vi "Pump waveplate.vi"(4 "Axis in":i32=3, 5 "Trigger rate warnings?":bool, 6 "appended array":dbl[][](array[numeric]), 7 "Trigger rate \nat 52.6 degrees":dbl, 8 "error in (no error)":errorcluster, 9 "Photon #":i32, 10 "Target trial \nlength (ms)":dbl, 11 "VISA Refnum in":refnum<visa-resource-name>) -> (0 "error out":errorcluster, 1 "WP Error":bool=TRUE, 2 "Current position (units)":dbl, 3 "VISA Refnum out":refnum<visa-resource-name>)   [LabVIEW 2013]
uses:
  <vilib>/imath/engines/lvmath2/RunTimeEngine/BuiltInFunctions/asin/NIMS_asin(C).vi
  <instcachedir>/0/NIMS_asin(C)_73B68F6B04904A8785972686F67E90FD.lvgen/NIMS_asin(C)_73B68F6B04904A8785972686F67E90FD_001.vi
  <vilib>/imath/engines/lvmath2/RunTimeEngine/NodeEndStatement/NIMS_NodeEndStatement_Output.vi
  <instcachedir>/0/NIMS_NodeEndStatement_Output_53EC0D466D134D7ABD903AC30B43404B.lvgen/NIMS_NodeEndStatement_Output_53EC0D466D134D7ABD903AC30B43404B_010.vi
  <instcachedir>/0/NIMS_NodeEndStatement_Output_53EC0D466D134D7ABD903AC30B43404B.lvgen/NIMS_NodeEndStatement_Output_53EC0D466D134D7ABD903AC30B43404B_001.vi
  <vilib>/imath/engines/lvmath2/RunTimeEngine/BuiltInFunctions/abs/NIMS_abs(signed).vi
  <instcachedir>/0/NIMS_abs(signed)_C4FCB8E6058B49B797C7C8D53CA5F6EC.lvgen/NIMS_abs(signed)_C4FCB8E6058B49B797C7C8D53CA5F6EC_000.vi
  <vilib>/imath/engines/lvmath2/RunTimeEngine/ErrorHandling/NIMS_Finalize Error.vi
  <instcachedir>/0/NIMS_NodeEndStatement_Output_53EC0D466D134D7ABD903AC30B43404B.lvgen/NIMS_NodeEndStatement_Output_53EC0D466D134D7ABD903AC30B43404B_009.vi
  <instcachedir>/0/NIMS_abs(signed)_C4FCB8E6058B49B797C7C8D53CA5F6EC.lvgen/NIMS_abs(signed)_C4FCB8E6058B49B797C7C8D53CA5F6EC_002.vi
panel:
  out "angle":dbl
  out "theta1":dbl
  out "t_ratio":dbl
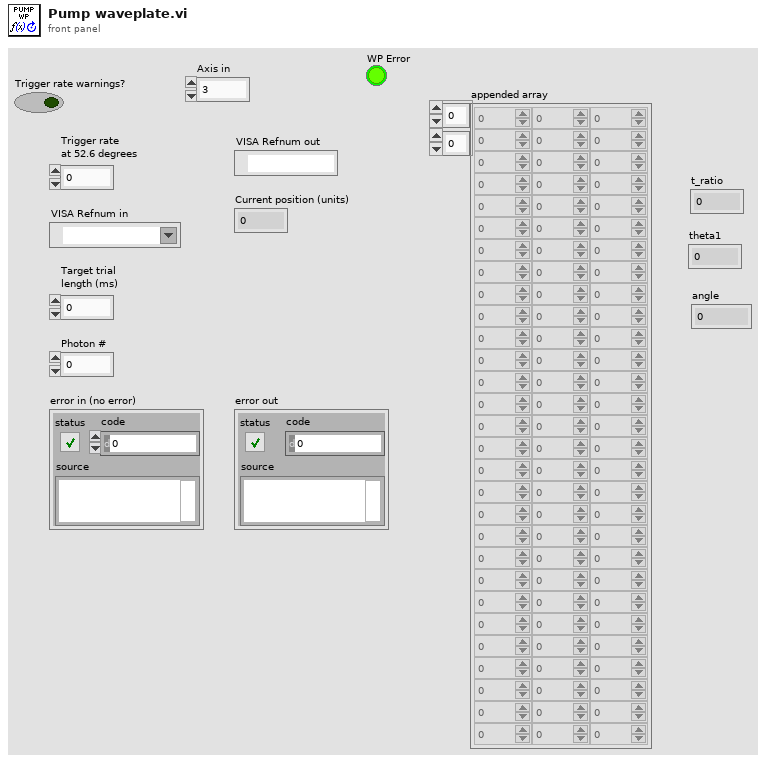
[diagram p1: front panel]
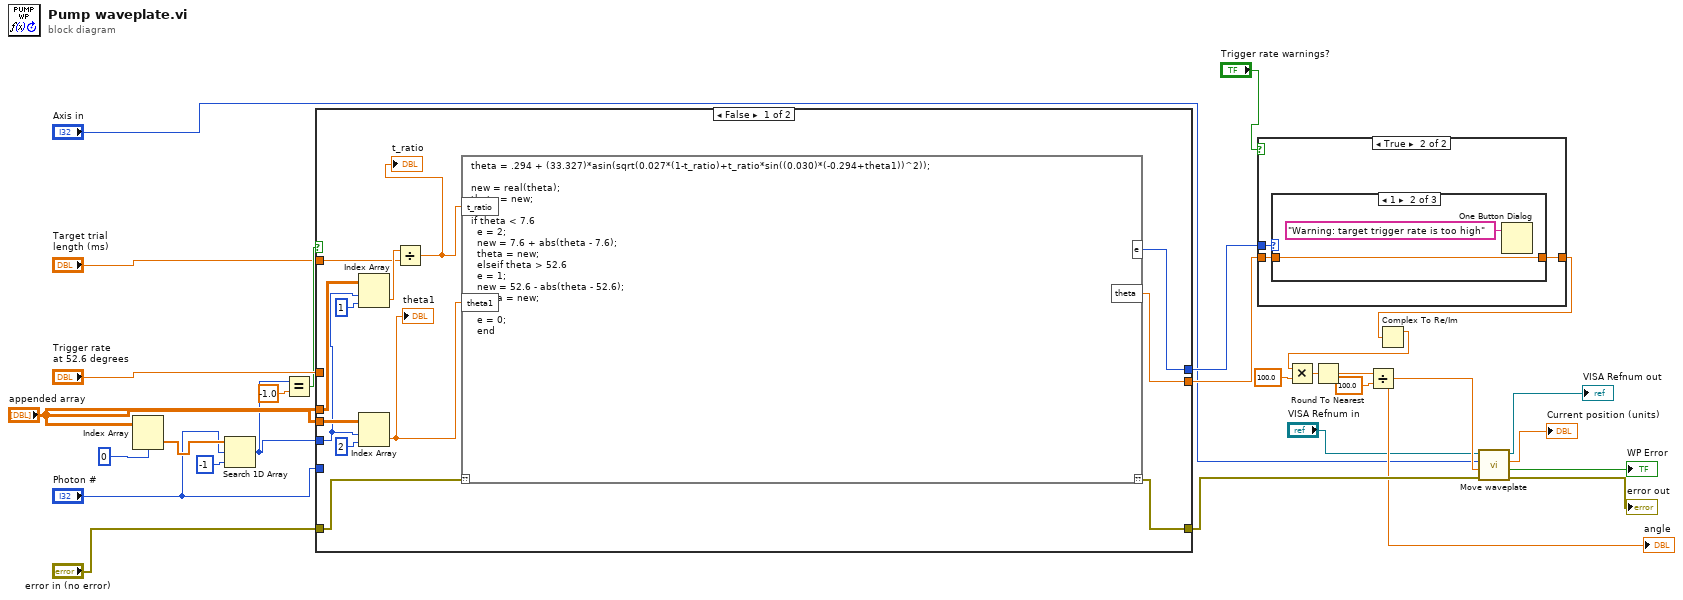
[diagram p0: block diagram]
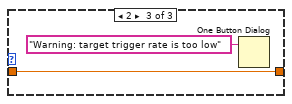
[diagram p4: hidden frame]
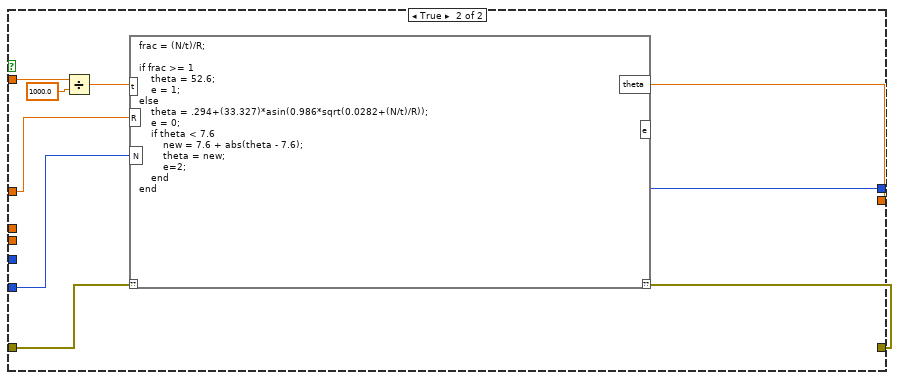
[diagram p5: hidden frame]
diagram:
  n1 = Index Array(array="appended array", index (col)=0 ("disabled index (col)")) -> (element=w24:dbl[])  [unwired: 1 in]
  n2 = Search 1D Array(1D array=w24, element="Photon #", start index (0)=-1) -> (index of element=w19:i32)
  n3 = Equal?(x=w19, y=-1.0) -> (x = y?=w21:bool)
  n4 = case shown="False" w21 {
    tunnel: "Trigger rate \nat 52.6 degrees" -> [_ w177]
    tunnel: [w29 w169] -> w16
    tunnel: [w32 w176] -> w27
    tunnel: "Target trial \nlength (ms)" -> [w33 w171]
    tunnel: "Photon #" -> [_ w175]
    tunnel: "error in (no error)" -> [w31 w174]
    tunnel: [w30 w173] -> w8
    tunnel: "appended array" -> [w36 _]
    tunnel: "appended array" -> [w35 _]
    tunnel: w19 -> [w34 _]
    frame False {
      n5 = Index Array(array=w35, index (row)=w34, index (col)=1 ("disabled index (col)")) -> (element=w39:dbl)
      n6 = Index Array(array=w36, index (row)=w34, index (col)=2 ("disabled index (col)")) -> (element=w38:dbl)
      "theta1" <- w38
      n7 = Divide(x=w39, y=w33) -> (x/y=w37:dbl)
      "t_ratio" <- w37
      n8 = mathscript code="theta = .294 + (33.327)*asin(sqrt(0.027*(1-t_ratio)+t_ratio*sin((0.030)*(-0.294+theta1))^2));\n\nnew = real(theta);\ntheta = new;\n\nif theta < 7.6\n  e = 2;\n  new = 7.6 + abs(theta - 7.6);\n  theta = new;\n  elseif theta > 52.6\n  e = 1;\n  new = 52.6 - abs(theta - 52.6);\n  theta = new;\n  else\n  e = 0;\n  end"("??"=w31, "t_ratio"=w37, "theta1"=w38) -> ("??"=w30:errorcluster, "e"=w32:i32, "theta"=w29:dbl)
    }
    frame True {
      n9 = Divide(x=w171, y=1000.0) -> (x/y=w170:dbl)
      n10 = mathscript code="frac = (N/t)/R;\n\nif frac >= 1\n    theta = 52.6;\n    e = 1;\nelse\n    theta = .294+(33.327)*asin(0.986*sqrt(0.0282+(N/t)/R));\n    e = 0;\n    if theta < 7.6\n        new = 7.6 + abs(theta - 7.6);\n        theta = new;\n        e=2;\n    end\nend"("??"=w174, "t"=w170, "R"=w177, "N"=w175) -> ("??"=w173:errorcluster, "e"=w176:i32, "theta"=w169:cdb)
    }
  }
  n11 = case shown="True" "Trigger rate warnings?" {
    tunnel: [w294 w297] -> w15
    tunnel: w16 -> [w294 w296]
    tunnel: w27 -> [_ w295]
    frame False {
    }
    frame True {
      n12 = case shown="1" w295 {
        tunnel: w296 -> [w298 w299 w301]
        tunnel: [w298 w299 w301] -> w297
        frame 0, Default {
        }
        frame 1 {
          n13 = One Button Dialog(message="Warning: target trigger rate is too high") -> ()  [unwired: 1 in, 1 out]
        }
        frame 2 {
          n14 = One Button Dialog(message="Warning: target trigger rate is too low") -> ()  [unwired: 1 in, 1 out]
        }
      }
    }
  }
  n15 = Complex To Re/Im(x + iy=w15) -> (x=w14:dbl)  [unwired: 1 out]
  n16 = Multiply(x=w14, y=100.0) -> (x*y=w12:dbl)
  n17 = Round To Nearest(number=w12) -> (nearest integer value=w11:dbl)
  n18 = Divide(x=w11, y=100.0) -> (x/y=w7:dbl)
  "angle" <- w7
  n19 = call "Move waveplate.vi"("error in (no error)"=w8, "Angle"=w7, "Axis in"="Axis in", "VISA Refnum in"="VISA Refnum in") -> ("error out"=→"error out":errorcluster, "WP Error"=→"WP Error":bool, "Current position (units)"=→"Current position (units)":dbl, "VISA Refnum out"=→"VISA Refnum out":refnum<visa-resource-name>)  [unwired: 4 in]
